vi "Next_CMDs.vi"(11 "MBCMDs":T1[](array[typedef]) {"Function Code" items=["Read Coils"=1, "Read Discrete Inputs"=2, "Read Holding Registers"=3, "Read Input Registers"=4, "Write Single Coil"=5, "Write Single Register"=6, "Read Exception Status"=7, "Write Multiple Coils"=15, "Write Multiple Registers"=16]}) -> (3 "MBCMD Out":T1[](array[typedef]) {"Function Code" items=["Read Coils"=1, "Read Discrete Inputs"=2, "Read Holding Registers"=3, "Read Input Registers"=4, "Write Single Coil"=5, "Write Single Register"=6, "Read Exception Status"=7, "Write Multiple Coils"=15, "Write Multiple Registers"=16]})   [LabVIEW 2020, in "ModBus Serial Master.lvlib"]
uses:
  ModBus Serial Master.lvlib
  DriverCommon/MB Modbus Command.ctl
  DriverCommon.lvlib
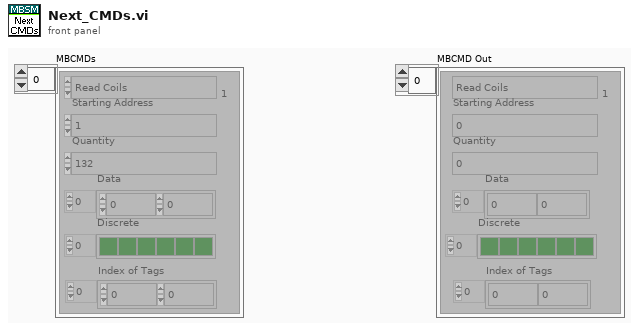
[diagram p1: front panel]
types:
  T1 = typedef "DriverCommon.lvlib/MB Modbus Command.ctl" = cluster{"Function Code":u8, "Starting Address":u16, "Quantity":u16, "Data":u16[], "Discrete":bool[], "Index of Tags":i32[]}
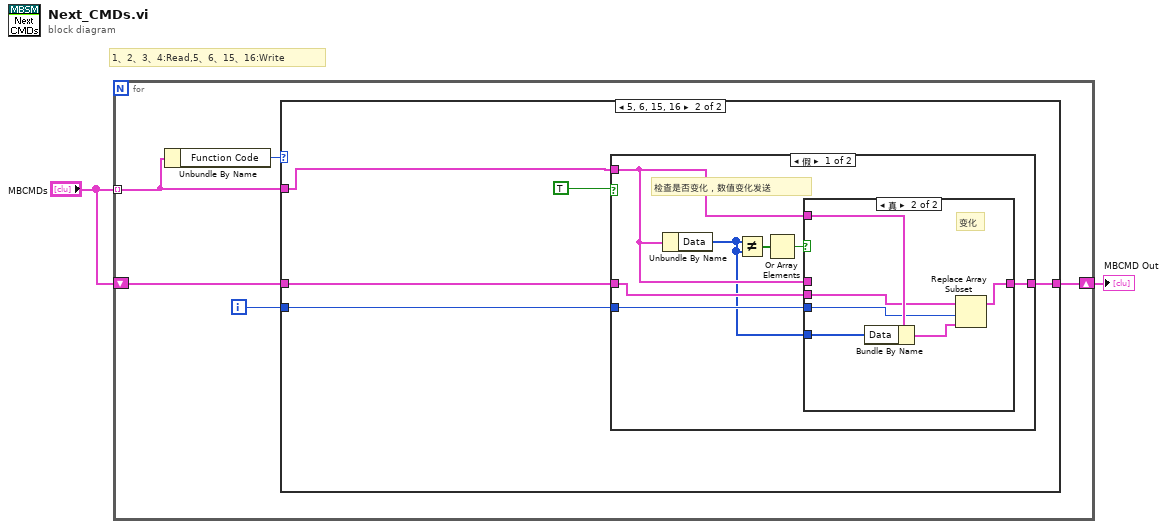
[diagram p0: block diagram]
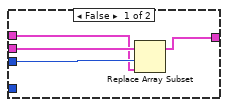
[diagram p3: hidden frame]
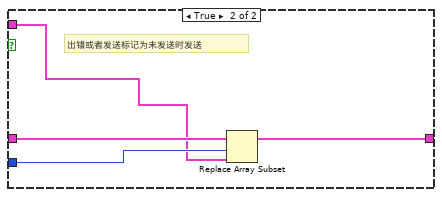
[diagram p4: hidden frame]
diagram:
  # "1、2、3、4:Read,5、6、15、16:Write"
  n1 = for {
    tunnel: "MBCMDs" -> [w6] mode=indexing
    shift-right: [w4] -> w2
    shift-left: "MBCMDs" -> [w5]
    i -> [w3]
    n2 = Unbundle By Name(w6) -> ("Function Code"=w7:u8)
    n3 = case shown="5, 6, 15, 16" w7 {
      tunnel: w6 -> [_ w13]
      tunnel: w5 -> [w8 w12]
      tunnel: [w8 w11] -> w4
      tunnel: w3 -> [_ w10]
      frame 1..4, Default {
      }
      frame 5, 6, 15, 16 {
        n4 = case shown="假" TRUE ("Enable") {
          tunnel: w13 -> [w15 w31]
          tunnel: w12 -> [w19 w34]
          tunnel: [w18 w33] -> w11
          tunnel: w10 -> [w16 w32]
          frame False {
            # "检查是否变化，数值变化发送"
            n5 = Unbundle By Name(w15) -> ("Data"=w14:u16[])
            n6 = Not Equal?(x=w14, y=w14) -> (x != y?=w17:bool[])
            n7 = Or Array Elements(Boolean array=w17) -> (logical OR=w20:bool)
            n8 = case shown="真" w20 {
              tunnel: w15 -> [_ w30]
              tunnel: w19 -> [w24 w28]
              tunnel: [w23 w27] -> w18
              tunnel: w16 -> [w22 w26]
              tunnel: w15 -> [w21 _]
              tunnel: w14 -> [_ w25]
              frame False {
                n9 = Replace Array Subset(array=w24, new element=w21, index=w22) -> (w23:T1[])
              }
              frame True {
                # "变化"
                n10 = Bundle By Name(cluster=w30, "Data"=w25) -> (w29:T1)
                n11 = Replace Array Subset(array=w28, new element=w29, index=w26) -> (w27:T1[])
              }
            }
          }
          frame True {
            # "出错或者发送标记为未发送时发送"
            n12 = Replace Array Subset(array=w34, new element=w31, index=w32) -> (w33:T1[])
          }
        }
      }
    }
  }
  "MBCMD Out" <- w2
